vi "OuterFunction.vi"() -> ()   [LabVIEW 2012]
uses:
  GlobalVariables_DIALMain.vi
panel:
  in  "User Comment":bool
  in  "Update Permissions":bool
  in  "Global Abort":bool
  in  "Tab Control":T1(tab)
  out "error IO":errorcluster
  out "LoopCounter":i32
  out "Permission Level":T2(ring)
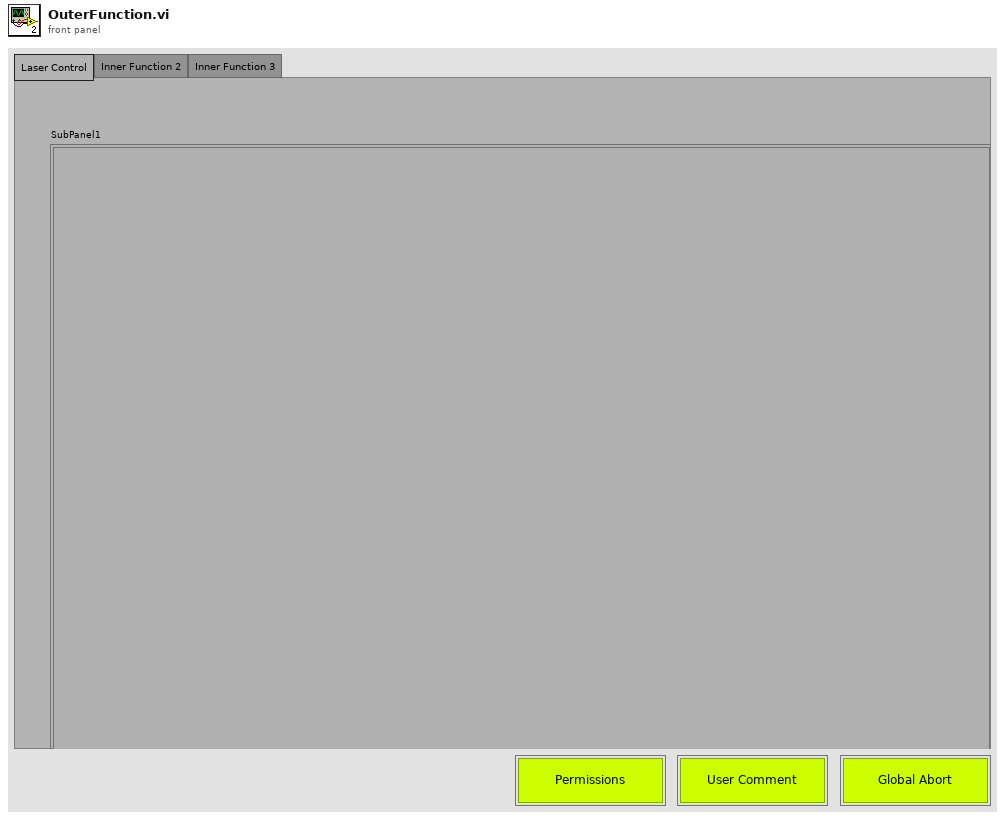
[diagram p1: front panel]
types:
  T1 = enum32{"Laser Control", "Inner Function 2", "Inner Function 3"}
  T2 = enum16{"Unset", "Operator", "Administrator", "Full"}
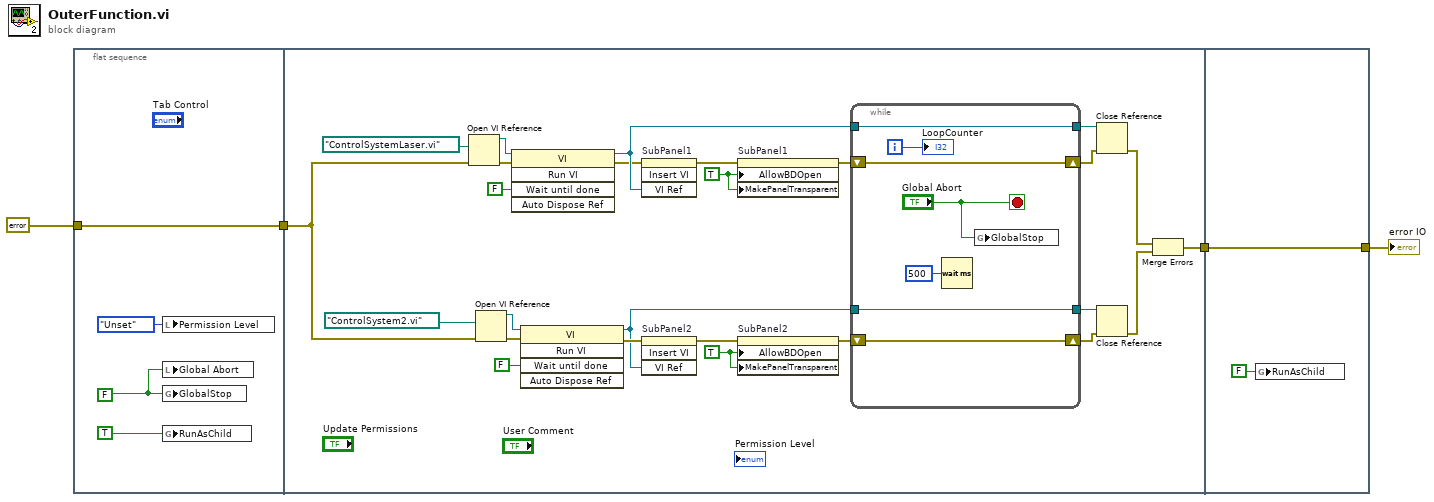
[diagram p0: block diagram]
diagram:
  n1 = flat-sequence {
    tunnel: errorcluster {"status"=FALSE, "code"=0, "source"=""} ("error in (no error)") -> [w8]
    tunnel: [w8] -> w3
    tunnel: w3 -> [w25]
    tunnel: [w13] -> w1
    tunnel: [w43] -> w2
    tunnel: w1 -> [w43]
    frame #0 {
      w6 = FALSE ("Global Stop")
      n2 = local write "Permission Level"(T2."Unset" ("Permission Level")) -> ()
      n3 = local write "Global Abort"(w6) -> ()
      n4 = global write "GlobalVariables_DIALMain.vi" "GlobalStop"(w6) -> ()
      n5 = global write "GlobalVariables_DIALMain.vi" "RunAsChild"(TRUE ("RunAsChild")) -> ()
    }
    frame #1 {
      w11 = TRUE ("Allow User to Open Diagram")
      w12 = TRUE ("Allow User to Open Diagram")
      n6 = Open VI Reference(vi path=path "ControlSystemLaser.vi", error in (no error)=w25) -> (vi reference=w33:refnum<vi>, error out=w32:errorcluster)  [unwired: 4 in]
      n7 = Open VI Reference(vi path=path "ControlSystem2.vi", error in (no error)=w25) -> (vi reference=w24:refnum<vi>, error out=w23:errorcluster)  [unwired: 4 in]
      n8 = invoke class="VI" method="Run VI"(reference=w33, error in=w32, "Wait until done"=FALSE ("Wait Until Done")) -> (reference out=w10:refnum<vi>, error out=w9:errorcluster)  [unwired: 2 in, 3 out]
      n9 = invoke class="VI" method="Run VI"(reference=w24, error in=w23, "Wait until done"=FALSE ("Wait Until Done")) -> (reference out=w18:refnum<vi>, error out=w21:errorcluster)  [unwired: 2 in, 3 out]
      n10 = invoke on="SubPanel1" class="SubPanel" method="Insert VI"(error in=w9, "VI Ref"=w10) -> (error out=w28:errorcluster)  [unwired: 2 in, 3 out]
      n11 = invoke on="SubPanel2" class="SubPanel" method="Insert VI"(error in=w21, "VI Ref"=w18) -> (error out=w20:errorcluster)  [unwired: 2 in, 3 out]
      n12 = property on="SubPanel1" class="SubPnl"(error in=w28, "AllowBDOpen"=w12, "MakePanelTransparent"=w12) -> (error out=w27:errorcluster)  [unwired: 1 in, 1 out]
      n13 = property on="SubPanel2" class="SubPnl"(error in=w20, "AllowBDOpen"=w11, "MakePanelTransparent"=w11) -> (error out=w19:errorcluster)  [unwired: 1 in, 1 out]
      n14 = while {
        tunnel: w10 -> [w41]
        tunnel: [w41] -> w30
        shift-right: [w40] -> w29
        shift-left: w27 -> [w40]
        shift-right: [w37] -> w16
        shift-left: w19 -> [w37]
        tunnel: w18 -> [w36]
        tunnel: [w36] -> w17
        i -> [w38]
        stop <- "Global Abort" stop-if-true
        n15 = Wait (ms)(milliseconds to wait=u32 500) -> ()  [unwired: 1 out]
        n16 = global write "GlobalVariables_DIALMain.vi" "GlobalStop"("Global Abort") -> ()
        "LoopCounter" <- w38
      }
      n17 = Close Reference(reference=w30, error in (no error)=w29) -> (error out=w15:errorcluster)
      n18 = Close Reference(reference=w17, error in (no error)=w16) -> (error out=w14:errorcluster)
      n19 = Merge Errors(w15, w14) -> (w13:errorcluster)
    }
    frame #2 {
      n20 = global write "GlobalVariables_DIALMain.vi" "RunAsChild"(FALSE ("RunAsChild")) -> ()
    }
  }
  "error IO" <- w2
